vi "Sollwerte vom GT übernehmen.vi"(5 "höchste Konzentration Teilkomponente":dbl, 7 "Gesamtkonzentration":dbl, 8 "error in (no error)":errorcluster caption="Fehler (Eingang, kein Fehler)", 9 "Einheit in String":string, 10 "DoIt":bool, 11 "Gasindex":i32) -> (0 "error out":errorcluster caption="Fehler (Ausgang)", 3 "Gasindex out":i32)   [LabVIEW 2020, in "Linearisierung v2.lvlib"]
uses:
  Linearisierung v2.lvlib
  Aktion Lin Daten aufarbeiten.ctl
  Gasteiler/Gasteiler.lvlib
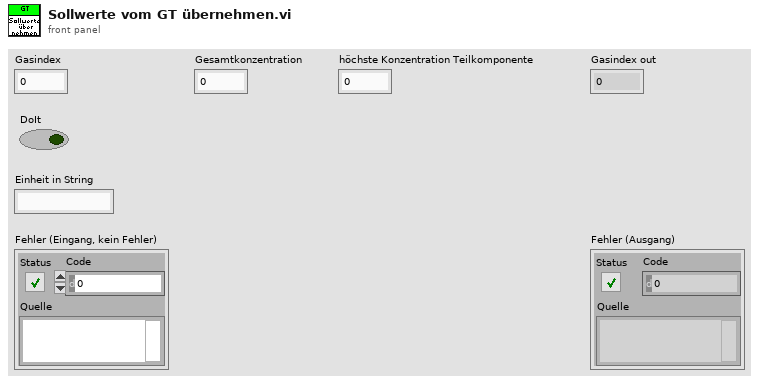
[diagram p1: front panel]
types:
  T1 = typedef "Linearisierung v2.lvlib/Aktion Lin Daten aufarbeiten.ctl" = enum16{"lesen", "Protkolldaten", "speichern", "laden", "EPA auswerten", "Tabelle schreiben", "Lin auswerten", "Tab init", "Stufentabelle", "EPA aktiviert", "Nachbehandlung laden", "Tabelle löschen", "Istwerte löschen", "Zeile löschen", "Zeile einfügen", "LIN aktiviert", "LIN/EPA aktiv laden", "EGAK Tab", "LIN übernehmen", "Tab init ohne Stufen"}
  T2 = typedef "Linearisierung v2.lvlib/Eingabetabelle.ctl" = string[][]
  T3 = typedef "Linearisierung v2.lvlib/Gasteiler.lvlib/Stufen Tabelle.ctl" = string[][]
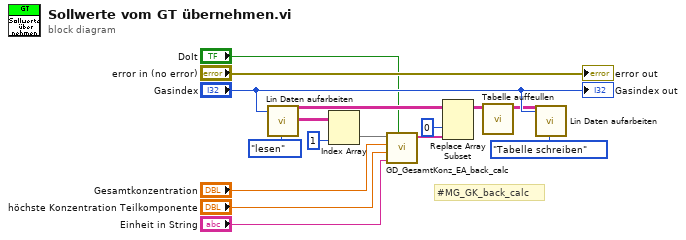
[diagram p0: block diagram]
diagram:
  # "#MG_GK_back_calc"
  n1 = call "Lin Daten aufarbeiten.vi"("Index (Seite)"="Gasindex", "Aktionen"=Aktion_Lin_Daten_aufarbeiten."lesen") -> ("Eingabetabelle"=w9:T2, "Stufen Tabelle"=w15:T3)  [unwired: 15 in, 9 out]
  n2 = Index Array(array=w15, index (col)=1 ("Deaktivierter Index (Spalte)")) -> (element=w6:string[])  [unwired: 1 in]
  n3 = call "GD_GesamtKonz_EA_back_calc.vi"("DoIt"="DoIt", "Einheit in String"="Einheit in String", "höchste Konzentration Teilkomponente"="höchste Konzentration Teilkomponente", "Gesamtkonzentration"="Gesamtkonzentration", "Stufentabelle (Eingang)"=w6) -> ("Sollwerte EA Tabelle (Ausgang)"=w5:string[])  [unwired: 6 in]
  n4 = Replace Array Subset(array=w9, new element=w5, index (col)=0 ("Deaktivierter Index (Spalte)")) -> (w11:T2)  [unwired: 1 in]
  n5 = call "Tabelle auffeullen.vi"("Neue Tabelle"=w11) -> ("Tabelle"=w8:string[][])  [unwired: 10 in]
  n6 = call "Lin Daten aufarbeiten.vi"("Eingabetabelle"=w8, "Index (Seite)"="Gasindex", "Aktionen"=Aktion_Lin_Daten_aufarbeiten."Tabelle schreiben") -> ()  [unwired: 14 in, 11 out]
  "error out" <- "error in (no error)"
  "Gasindex out" <- "Gasindex"
